vi "test8-AsyncMessageWithoutReply_API.vi"(8 "error in (no error)":errorcluster, 11 "TestCase in":refnum<class "testcase-CSMMessage.lvclass">) -> (0 "error out":errorcluster, 3 "TestCase out":refnum<class "testcase-CSMMessage.lvclass">)   [LabVIEW 2017, in "testcase-CSMMessage.lvclass"]
uses:
  testcase-CSMMessage.lvclass
  7412589e-de49-4983-aece-358686b48526.vi
  <vilib>/addons/_JKI Toolkits/VI Tester/TestCase.llb/TestCase.lvclass
  src/user.lib/_NEVSTOP/Communicable State Machine(CSM)/Communicable State Machine.lvlib
  C:/Program Files (x86)/National Instruments/LabVIEW 2017/vi.lib/addons/_JKI Toolkits/VI Tester/TestCase.llb/TestCase.lvclass
panel:
  out "Loop count":i32
  out "debug message":string
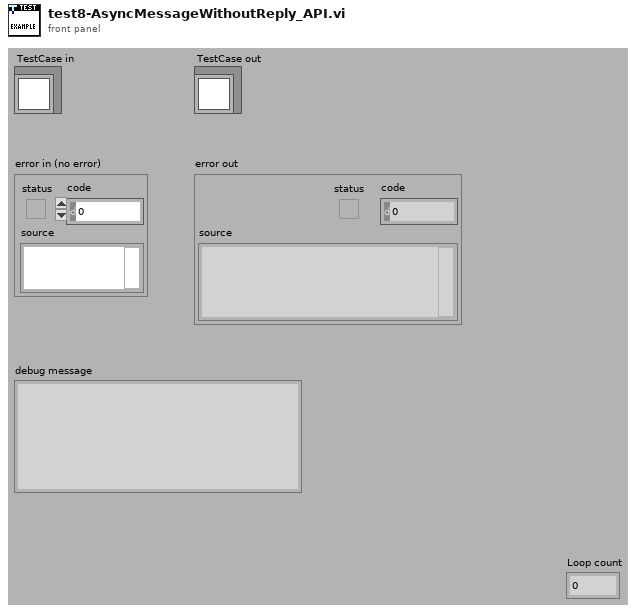
[diagram p1: front panel]
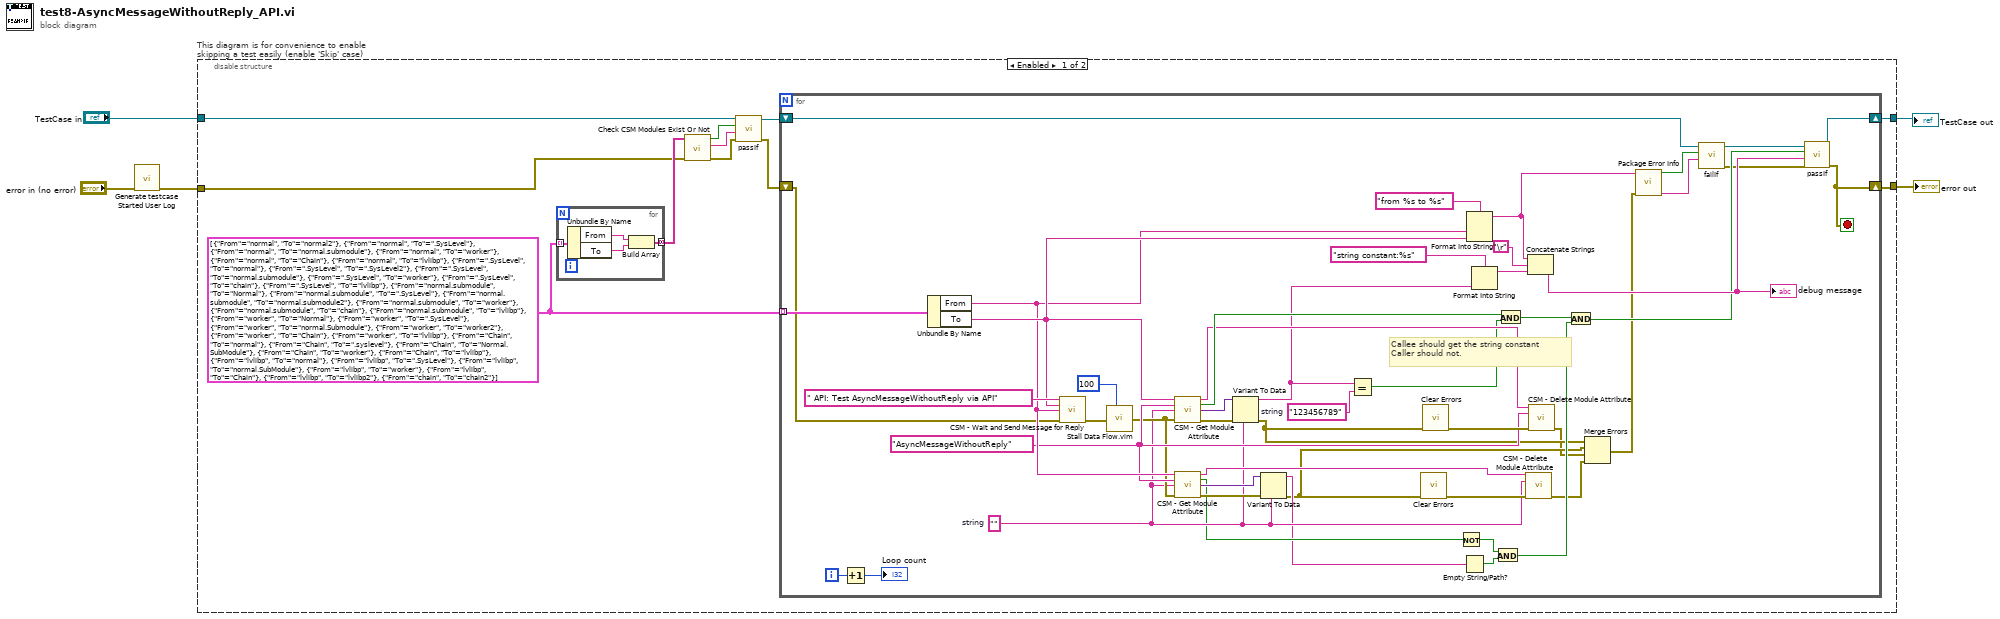
[diagram p0: block diagram]
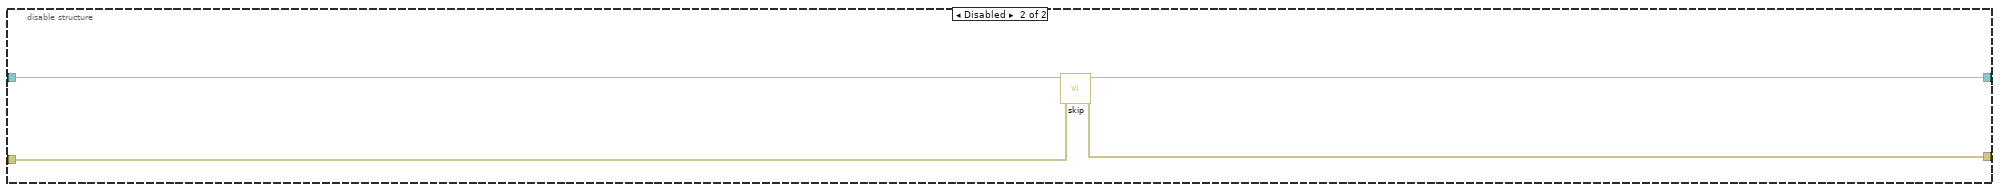
[diagram p2: hidden frame]
diagram:
  n1 = call "Generate testcase Started User Log.vi"("Error In"="error in (no error)") -> ("error out"=w1:errorcluster)  [unwired: 10 in]
  n2 = disable-structure "This diagram is for convenience to enable skipping a test easily (enable 'Skip' case)" shown="Enabled" {
    disable-tunnel: "TestCase in" -> [w9 w73]
    disable-tunnel: [w7 w71] -> w2
    disable-tunnel: [w6 w72] -> w4
    disable-tunnel: w1 -> [w10 w70]
    frame Enabled {
      w12 = cluster{"From":string, "To":string}[] [{"From"="normal", "To"="normal2"}, {"From"="normal", "To"=".SysLevel"}, {"From"="normal", "To"="normal.submodule"}, {"From"="normal", "To"="worker"}, {"From"="normal", "To"="Chain"}, {"From"="normal", "To"="lvlibp"}, {"From"=".SysLevel", "To"="normal"}, {"From"=".SysLevel", "To"=".SysLevel2"}, {"From"=".SysLevel", "To"="normal.submodule"}, {"From"=".SysLevel", "To"="worker"}, {"From"=".SysLevel", "To"="chain"}, {"From"=".SysLevel", "To"="lvlibp"}, {"From"="normal.submodule", "To"="Normal"}, {"From"="normal.submodule", "To"=".SysLevel"}, {"From"="normal.submodule", "To"="normal.submodule2"}, {"From"="normal.submodule", "To"="worker"}, {"From"="normal.submodule", "To"="chain"}, {"From"="normal.submodule", "To"="lvlibp"}, {"From"="worker", "To"="Normal"}, {"From"="worker", "To"=".SysLevel"}, {"From"="worker", "To"="normal.Submodule"}, {"From"="worker", "To"="worker2"}, {"From"="worker", "To"="Chain"}, {"From"="worker", "To"="lvlibp"}, {"From"="Chain", "To"="normal"}, {"From"="Chain", "To"=".syslevel"}, {"From"="Chain", "To"="Normal.SubModule"}, {"From"="Chain", "To"="worker"}, {"From"="Chain", "To"="lvlibp"}, {"From"="lvlibp", "To"="normal"}, {"From"="lvlibp", "To"=".SysLevel"}, {"From"="lvlibp", "To"="normal.SubModule"}, {"From"="lvlibp", "To"="worker"}, {"From"="lvlibp", "To"="Chain"}, {"From"="lvlibp", "To"="lvlibp2"}, {"From"="chain", "To"="chain2"}]
      n3 = for {
        tunnel: w12 -> [w20] mode=indexing
        tunnel: [w17] -> w15 mode=concatenating
        n4 = Unbundle By Name(w20) -> ("From"=w19:string, "To"=w18:string)
        n5 = Build Array(w19, w18) -> (w17:string[])
      }
      n6 = call "Check CSM Modules Exist Or Not.vi"("error in"=w10, "CSM names in"=w15) -> ("error out"=w13:errorcluster, "Debug string"=w14:string, "All Modules Exist?"=w16:bool)  [unwired: 7 in]
      n7 = call-dynamic "passIf.vi"("error in (no error)"=w13, "message (\"\")"=w14, "pass"=w16, "TestCase in"=w9) -> ("error out"=w11:errorcluster, "TestCase out"=w8:refnum<class "testcase-CSMMessage.lvclass">)  [unwired: 6 in]
      n8 = for {
        tunnel: w12 -> [w64] mode=indexing
        shift-right: [w69] -> w7
        shift-left: w8 -> [w26]
        shift-right: [w56] -> w6
        shift-left: w11 -> [w21]
        i -> [w36]
        stop <- w56 stop-if-true
        w53 = "123456789"  # string
        w44 = ""  # string
        w50 = "AsyncMessageWithoutReply" ("State With Arguments")
        # "Callee should get the string constant\nCaller should not."
        n9 = Increment(x=w36) -> (x+1=→"Loop count":i32)
        n10 = Unbundle By Name(w64) -> ("From"=w51:string, "To"=w55:string)
        n11 = call "CSM - Wait and Send Message for Reply.vi"("State"=" API: Test AsyncMessageWithoutReply via API", "Arguments (\"\")"=w55, "Target Module"=w51, "Error In (No Error)"=w21) -> ("error out"=w34:errorcluster)  [unwired: 8 in, 3 out]
        n12 = call "Stall Data Flow.vim"("value in"=w34, "milliseconds to wait"=u32 100) -> ("value out"=w49:errorcluster)  [unwired: 1 out]
        n13 = call "CSM - Get Module Attribute.vi"("CSM Name"=w55, "Attribute"=w50, "Default Value (Empty Variant)"=w44, "Error In"=w49) -> ("CSM Name (Dup)"=w62:string, "Found"=w65:bool, "Value"=w66:variant, "error out"=w67:errorcluster)  [unwired: 7 in, 1 out]
        n14 = call "CSM - Get Module Attribute.vi"("CSM Name"=w51, "Attribute"=w50, "Default Value (Empty Variant)"=w44, "Error In"=w49) -> ("CSM Name (Dup)"=w45:string, "Found"=w43:bool, "Value"=w46:variant, "error out"=w48:errorcluster)  [unwired: 7 in, 1 out]
        n15 = Variant To Data(error in=w67, type=w44, Variant=w66) -> (data=w52:string, error out=w32:errorcluster)
        n16 = Variant To Data(error in=w48, type=w44, Variant=w46) -> (data=w42:string, error out=w31:errorcluster)
        n17 = Equal?(x=w52, y=w53) -> (x = y?=w54:bool)
        n18 = call <vilib>:"Clear Errors.vi"("error in (no error)"=w31) -> ("error out"=w47:errorcluster)  [unwired: 5 in, 1 out]
        n19 = call <vilib>:"Clear Errors.vi"("error in (no error)"=w32) -> ("error out"=w57:errorcluster)  [unwired: 5 in, 1 out]
        n20 = Not(x=w43) -> (.not. x?=w39:bool)
        n21 = Empty String/Path?(string/path=w42) -> (empty?=w41:bool)
        n22 = Format Into String(format string="from %s to %s", w51, w55) -> (resulting string=w22:string)  [unwired: 2 in, 1 out]
        n23 = Format Into String(format string="string constant:%s", w52) -> (resulting string=w61:string)  [unwired: 2 in, 1 out]
        n24 = And(x=w39, y=w41) -> (x .and. y?=w37:bool)
        n25 = And(x=w65, y=w54) -> (x .and. y?=w40:bool)
        n26 = call "CSM - Delete Module Attribute.vi"("CSM Name"=w45, "Attribute"=w44, "Error In"=w47) -> ("error out"=w29:errorcluster)  [unwired: 9 in, 3 out]
        n27 = Concatenate Strings(w22, "\r", w61) -> (w59:string)
        "debug message" <- w59
        n28 = call "CSM - Delete Module Attribute.vi"("CSM Name"=w62, "Attribute"=w50, "Error In"=w57) -> ("error out"=w30:errorcluster)  [unwired: 9 in, 3 out]
        n29 = And(x=w40, y=w37) -> (x .and. y?=w38:bool)
        n30 = Merge Errors(w32, w31, w30, w29) -> (w23:errorcluster)
        n31 = call "Package Error Info.vi"("error in"=w23, "String in"=w22) -> ("packed error info out"=w27:string, "error status"=w28:bool)  [unwired: 8 in]
        n32 = call-dynamic "failIf.vi"("message (\"\")"=w27, "fail"=w28, "TestCase in"=w26) -> ("error out"=w24:errorcluster, "TestCase out"=w25:refnum<class "testcase-CSMMessage.lvclass">)  [unwired: 7 in]
        n33 = call-dynamic "passIf.vi"("error in (no error)"=w24, "message (\"\")"=w59, "pass"=w38, "TestCase in"=w25) -> ("error out"=w56:errorcluster, "TestCase out"=w69:refnum<class "testcase-CSMMessage.lvclass">)  [unwired: 6 in]
      }
    }
    frame Disabled {
      # "skip test result while test is under development"
      n34 = call <vilib>:"skip.vi"("error in (no error)"=w70, "TestCase in"=w73) -> ("error out"=w72:errorcluster, "TestCase out"=w71:refnum<class "testcase-CSMMessage.lvclass">)  [unwired: 8 in]
    }
  }
  "error out" <- w4
  "TestCase out" <- w2
